vi "GetMyIPAddress.vi"(2 "Port":u32=5000, 3 "Format":T1(ring)) -> (0 "URI":string="http://192.168.1.8")   [LabVIEW 2013]
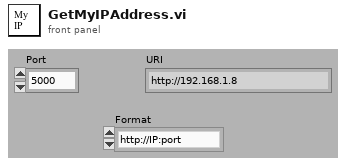
[diagram p1: front panel]
types:
  T1 = enum16{"http://IP:port", "http://IP", "IP:port", "IP only"}
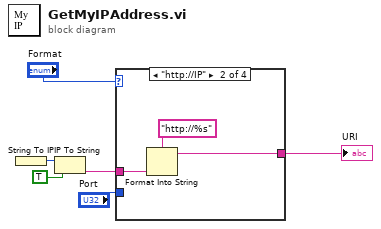
[diagram p0: block diagram]
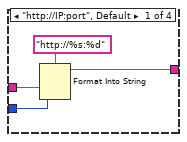
[diagram p2: hidden frame]
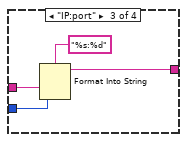
[diagram p3: hidden frame]
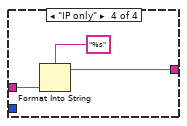
[diagram p4: hidden frame]
diagram:
  n1 = String To IP() -> (0:w3:u32)  [unwired: 1 in]
  n2 = IP To String(1:TRUE ("dot notation? (F)"), 2:w3) -> (0:w4:string)
  n3 = case shown="\"http://IP\"" "Format" {
    tunnel: w4 -> [w9 w12 w16 w19]
    tunnel: "Port" -> [w8 _ w14 _]
    tunnel: [w7 w11 w15 w18] -> w6
    frame "http://IP:port", Default {
      n4 = Format Into String(format string="http://%s:%d", w9, w8) -> (resulting string=w7:string)  [unwired: 2 in, 1 out]
    }
    frame "http://IP" {
      n5 = Format Into String(format string="http://%s", w12) -> (resulting string=w11:string)  [unwired: 2 in, 1 out]
    }
    frame "IP:port" {
      n6 = Format Into String(format string="%s:%d", w16, w14) -> (resulting string=w15:string)  [unwired: 2 in, 1 out]
    }
    frame "IP only" {
      n7 = Format Into String(format string="%s", w19) -> (resulting string=w18:string)  [unwired: 2 in, 1 out]
    }
  }
  "URI" <- w6
